vi "Commit NVMEM for Session.vi"(8 "error in (no error)":errorcluster, 11 "SLSC Interface in":refnum<class "SLSC Interface.lvclass">) -> (0 "error out":errorcluster, 3 "SLSC Interface out":refnum<class "SLSC Interface.lvclass">)   [LabVIEW 2016, in "SLSC Interface.lvclass"]
uses:
  SLSC Interface.lvclass
  nvmem type.ctl
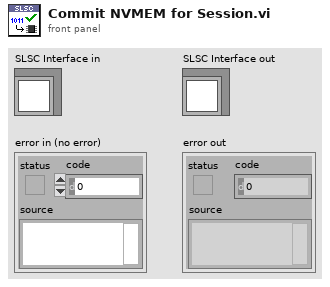
[diagram p1: front panel]
types:
  T1 = typedef "SLSC Interface.lvclass/nvmem type.ctl" = enum16{"area", "device", "session"}
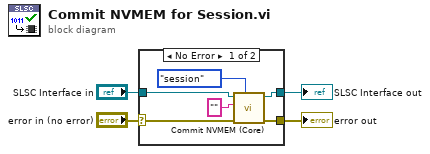
[diagram p0: block diagram]
diagram:
  n1 = case shown="No Error" "error in (no error)" {
    selector: "error in (no error)" -> [w6 w12]
    tunnel: [w5 w12] -> w3
    tunnel: [w9 w11] -> w1
    tunnel: "SLSC Interface in" -> [w10 w11]
    frame No Error {
      n2 = call "Commit NVMEM (Core).vi"("nvmem type"=nvmem_type."session", "error in (no error)"=w6, "resources"="", "SLSC Interface in"=w10) -> ("error out"=w5:errorcluster, "SLSC Interface out"=w9:refnum<class "SLSC Interface.lvclass">)  [unwired: 6 in]
    }
    frame Error {
    }
  }
  "error out" <- w3
  "SLSC Interface out" <- w1
